vi "reassemble_data.vi"(8 "Checksum":dbl, 9 "Interleaved 8bit Array":u8[](array[numeric]) format="%x", 11 "LSB First":bool=TRUE) -> (1 "reassembled 16 bit":u16[](array[numeric]) format="%x", 4 "MSB":u16[](array[numeric]) format="%x", 6 "LSB":u16[](array[numeric]) format="%x")   [LabVIEW 2012]
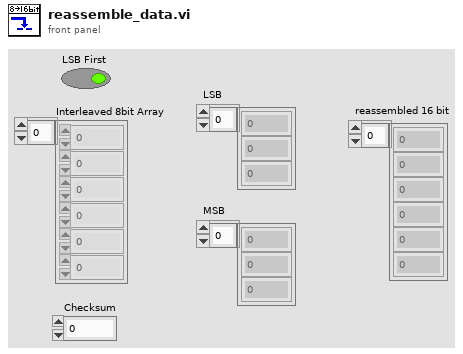
[diagram p1: front panel]
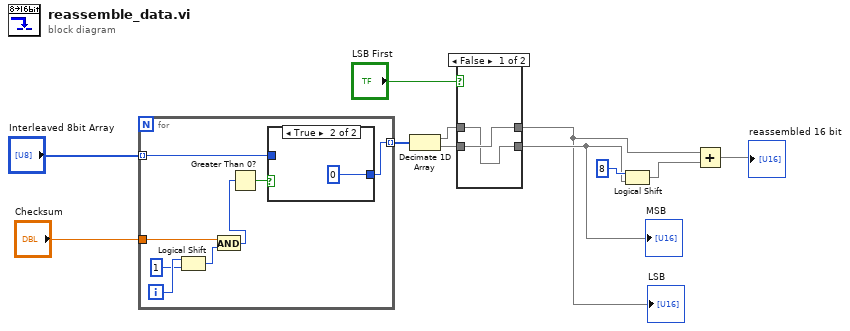
[diagram p0: block diagram]
diagram:
  n1 = for {
    tunnel: "Interleaved 8bit Array" -> [w14] mode=indexing
    tunnel: "Checksum" -> [w16]
    tunnel: [w15] -> w6 mode=indexing
    i -> [w19]
    n2 = Logical Shift(y=w19, x=1) -> (x << y=w17:i32)
    n3 = And(x=w16, y=w17) -> (x .and. y?=w12:i32)
    n4 = Greater Than 0?(x=w12) -> (x > 0?=w13:bool)
    n5 = case shown="True" w13 {
      tunnel: [w20 0] -> w15
      tunnel: w14 -> [w20 _]
      frame False {
      }
      frame True {
      }
    }
  }
  n6 = Decimate 1D Array(w6) -> (w2:i32[], w4:i32[])
  n7 = case shown="False" "LSB First" {
    tunnel: [w22 w25] -> w5
    tunnel: w4 -> [w23 w25]
    tunnel: [w23 w24] -> w3
    tunnel: w2 -> [w22 w24]
    frame False {
    }
    frame True {
    }
  }
  "LSB" <- w3
  "MSB" <- w5
  n8 = Logical Shift(y=i16 8, x=w5) -> (x << y=w10:i32[])
  n9 = Add(x=w3, y=w10) -> (x+y=→"reassembled 16 bit":i32[])
